vi "Write Bounds.vi"(5 "Bounds":T1, 9 "GObject in":refnum<class "GObject.lvclass">) -> (3 "GObject out":refnum<class "GObject.lvclass">)   [LabVIEW 2014, in "GObject.lvclass"]
uses:
  GObject.lvclass
  <vilib>/Utility/miscctls.llb/LVBoundsTypeDef.ctl
  GObject.lvclass/GObject.ctl
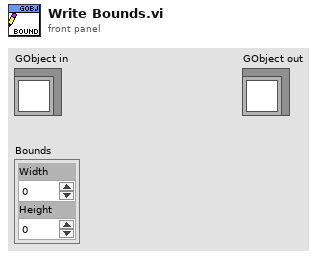
[diagram p1: front panel]
types:
  T1 = typedef "LVBoundsTypeDef.ctl" = cluster{"Width":u32, "Height":u32}
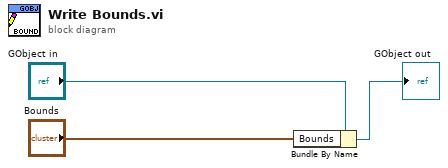
[diagram p0: block diagram]
diagram:
  n1 = Bundle By Name(cluster="GObject in", "Bounds"="Bounds") -> (→"GObject out":refnum<class "GObject.lvclass">)
